vi "Marshal.vi"(8 "error in (no error)":errorcluster, 11 "int32 in":refnum<class "bool.lvclass">) -> (0 "error out":errorcluster, 2 "Buffer":u8[](array[numeric]), 3 "int32 out":refnum<class "bool.lvclass">)   [LabVIEW 2020, in "Protobuf RAW.lvlib" / "bool.lvclass"]
uses:
  bool.lvclass
  bool.lvclass/bool.ctl
  4736b2cc-328e-48c1-834c-9aec0f57f3c9.vi
  4736b2cc-328e-48c1-834c-9aec0f57f3c9.vi/0f065a35-b637-42bd-ae45-04c3465bdb97.vi
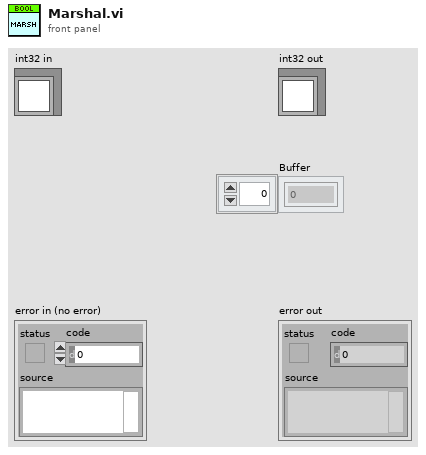
[diagram p1: front panel]
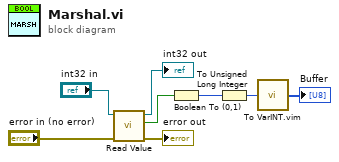
[diagram p0: block diagram]
diagram:
  n1 = call "Read Value.vi"("error in (no error)"="error in (no error)", "int32 in"="int32 in") -> ("error out"=→"error out":errorcluster, "Value"=w1:bool, "int32 out"=→"int32 out":refnum<class "bool.lvclass">)  [unwired: 7 in]
  n2 = Boolean To (0,1)(Boolean=w1) -> (0, 1=w7:i16)
  n3 = To Unsigned Long Integer(number=w7) -> (unsigned 32bit integer=w5:u32)
  n4 = call "To VarINT.vim"("Integer"=w5) -> ("LEB128"=→"Buffer":u8[])
